vi "Register gRPC Server.vi"(8 "error in (no error)":errorcluster, 10 "gRPC ID":T1, 11 "Plugin Manager in":refnum<class "CIFPluginManager.lvclass">) -> (0 "error out":errorcluster, 3 "Plugin Manager out":refnum<class "CIFPluginManager.lvclass">)   [LabVIEW 2021, in "CIFPluginManager.lvclass"]
uses:
  CIFPluginManager.lvclass
  <vilib>/gRPC/LabVIEW gRPC Library/Shared/grpcId.ctl
  CIF_Manager_server/RPC Service/Manager/Manager.lvclass
  C:/Program Files/National Instruments/LabVIEW 2021/vi.lib/gRPC/LabVIEW gRPC Servicer/ServiceBase/ServiceBase.lvclass
  CIFPluginManager.lvclass/CIFPluginManager.ctl
  CIF_Manager_server/CIF_Manager_server.lvlib
  <vilib>/gRPC/LabVIEW gRPC Library/grpc-lvsupport-release.lvlib
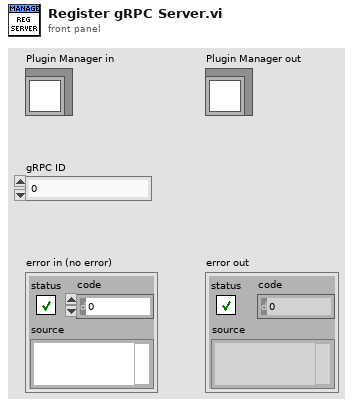
[diagram p1: front panel]
types:
  T1 = typedef "grpc-lvsupport-release.lvlib/grpcId.ctl" = u64
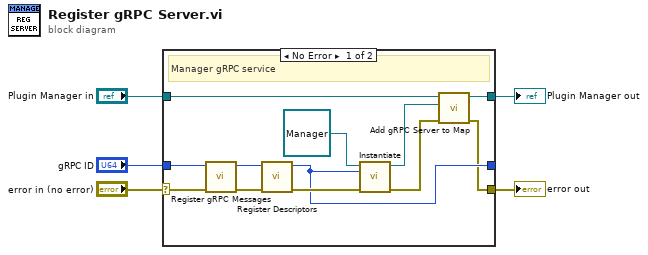
[diagram p0: block diagram]
diagram:
  n1 = case shown="No Error" "error in (no error)" {
    selector: "error in (no error)" -> [w15 w20]
    tunnel: [w6 w20] -> w4
    tunnel: [w11 w19] -> w2
    tunnel: "Plugin Manager in" -> [w12 w19]
    tunnel: "gRPC ID" -> [w14 w18]
    tunnel: [w7 w18] -> _
    frame No Error {
      # "Manager gRPC service"
      n2 = call "Register gRPC Messages.vi"("error in (no error)"=w15, "gRPC ID"=w14) -> ("error out"=w16:errorcluster, "gRPC ID Out"=w17:T1)  [unwired: 8 in]
      n3 = call "Register Descriptors.vi"("error in (no error)"=w16, "gRPC ID"=w17) -> ("error out"=w13:errorcluster, "gRPC ID Out"=w7:T1)  [unwired: 8 in]
      n4 = call-dynamic "Instantiate.vi"("error in"=w13, "gRPCid"=w7, "iService"=refnum<class "Manager.lvclass"> refnum ("CIF_Plugin_Core_server.lvlib:PluginCore.lvclass")) -> ("error out"=w9:errorcluster, "iService"=w8:refnum<class "Manager.lvclass">)  [unwired: 7 in]
      n5 = call "Add gRPC Server to Map.vi"("error in (no error)"=w9, "gRPC Server Class"=w8, "Plugin Manager in"=w12) -> ("error out"=w6:errorcluster, "Plugin Manager out"=w11:refnum<class "CIFPluginManager.lvclass">)  [unwired: 7 in]
    }
    frame Error {
    }
  }
  "error out" <- w4
  "Plugin Manager out" <- w2
